vi "Set Pin Status_UI Actor.vi"(6 "Valor pin":string(combo), 8 "error in (no error)":errorcluster, 9 "PIN":i32, 10 "CH":i32, 11 "UI Actor in":refnum<class "UI Actor.lvclass">) -> (0 "error out":errorcluster, 3 "UI Actor out":refnum<class "UI Actor.lvclass">)   [LabVIEW 2020, in "UI Actor.lvlib" / "UI Actor.lvclass"]
uses:
  UI Actor.lvclass
  UI Actor.lvclass/UI Actor.ctl
  Abstract/Serial Device/Serial Device.lvclass
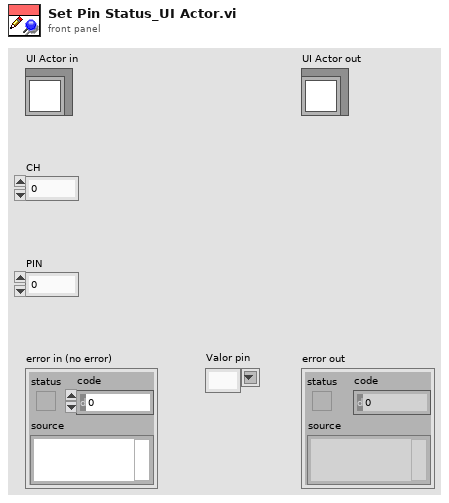
[diagram p1: front panel]
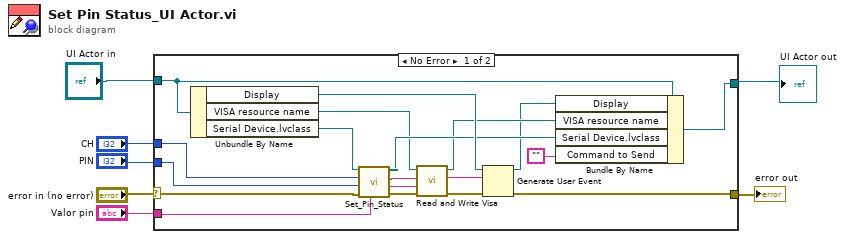
[diagram p0: block diagram]
diagram:
  n1 = case shown="No Error" "error in (no error)" {
    selector: "error in (no error)" -> [w10 w28]
    tunnel: [w21 w28] -> w6
    tunnel: [w22 w27] -> w4
    tunnel: "UI Actor in" -> [w23 w27]
    tunnel: "CH" -> [w26 _]
    tunnel: "PIN" -> [w25 _]
    tunnel: "Valor pin" -> [w24 _]
    frame No Error {
      n2 = Unbundle By Name(w23) -> ("Display"=w16:refnum<user-event>, "VISA resource name"=w9:refnum<visa-resource-name>, "Serial Device.lvclass"=w17:refnum<class "Serial Device.lvclass">)
      n3 = call-dynamic "Set_Pin_Status.vi"("Valor pin"=w24, "error in (no error)"=w10, "PIN"=w25, "CH"=w26, "Serial Device in"=w17) -> ("error out"=w19:errorcluster, "Expected Response"=w11:string, "Command to Send"=w12:string, "Serial Device out"=w15:refnum<class "Serial Device.lvclass">)  [unwired: 3 in]
      n4 = call "Read and Write Visa.vi"("error in (no error)"=w19, "Expected Response"=w11, "Command to Send"=w12, "VISA Refnum in"=w9) -> ("error out"=w18:errorcluster, "Expected Response out"=w20:string, "VISA Refnum out"=w14:refnum<visa-resource-name>)  [unwired: 5 in]
      n5 = Generate User Event(user event=w16, event data cluster=w20, error in=w18) -> (user event out=w13:refnum<user-event>, error out=w21:errorcluster)  [unwired: 1 in]
      n6 = Bundle By Name(cluster=w23, "Display"=w13, "VISA resource name"=w14, "Serial Device.lvclass"=w15, "Command to Send"="") -> (w22:refnum<class "UI Actor.lvclass">)
    }
    frame Error {
    }
  }
  "error out" <- w6
  "UI Actor out" <- w4
